vi "Start Frequency Scan.vi"(8 "error in (no error)":errorcluster, 10 "reset time (true)":bool=TRUE, 11 "VI Probe in":refnum<class "PL MKS VI Probe.lvclass">) -> (0 "error out":errorcluster, 3 "VI Probe out":refnum<class "PL MKS VI Probe.lvclass">)   [LabVIEW 2015, in "PL MKS VI Probe.lvclass"]
doc: "Starts frequency scan."
uses:
  PL MKS VI Probe.lvclass
  PL MKS VI Probe.lvclass/PL MKS VI Probe.ctl
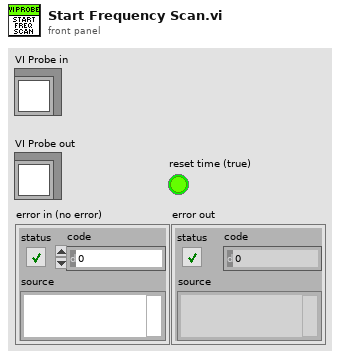
[diagram p1: front panel]
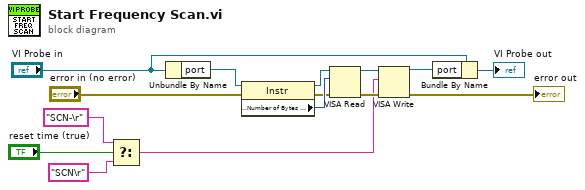
[diagram p0: block diagram]
diagram:
  n1 = Select(t="SCN-\r" ("format string"), s="reset time (true)", f="SCN\r" ("format string")) -> (s? t:f=w1:string)
  n2 = Unbundle By Name("VI Probe in") -> ("port"=w5:refnum<visa-resource-name>)
  n3 = property class="Instr"(reference=w5, error in="error in (no error)") -> (reference out=w11:refnum<visa-resource-name>, error out=w8:errorcluster, "Serial Settings:Number of Bytes at Serial Port"=w12:u32)
  n4 = VISA Read(VISA resource name=w11, byte count=w12, error in (no error)=w8) -> (VISA resource name out=w10:refnum<visa-resource-name>, error out=w9:errorcluster)  [unwired: 2 out]
  n5 = VISA Write(VISA resource name=w10, write buffer=w1, error in (no error)=w9) -> (VISA resource name out=w4:refnum<visa-resource-name>, error out=→"error out":errorcluster)  [unwired: 1 out]
  n6 = Bundle By Name(cluster="VI Probe in", "port"=w4) -> (→"VI Probe out":refnum<class "PL MKS VI Probe.lvclass">)
